vi "old_HWGlobalsToObject.vi"(7 "Select Layout":refnum<vi>, 8 "error in (no error)":errorcluster, 10 "Master AO Channel":T1, 11 "NI Card in":refnum<class "NI Card.lvclass">) -> (0 "error out":errorcluster, 3 "NI Card out":refnum<class "NI Card.lvclass">)   [LabVIEW 2013, in "NI Card.lvclass"]
uses:
  NI Card.lvclass
  NI Card.lvclass/NI Card.ctl
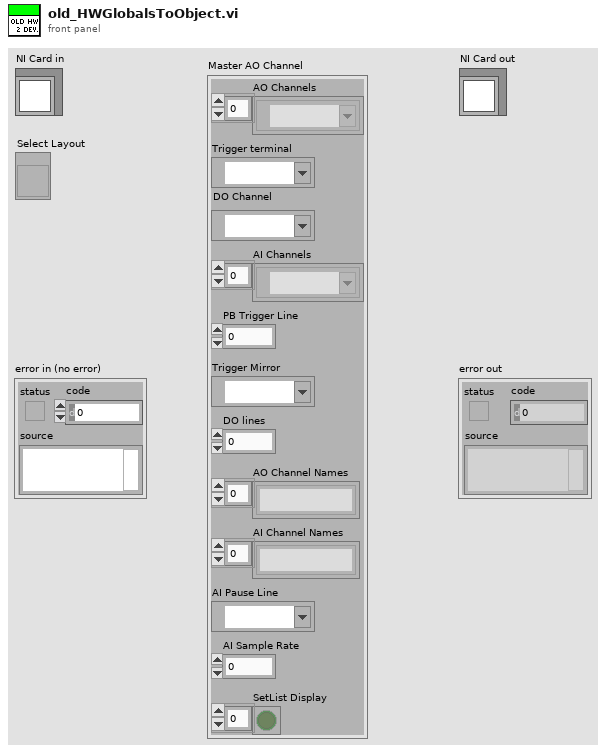
[diagram p1: front panel]
types:
  T1 = cluster{"AO Channels":refnum<k21>[], "Trigger terminal":tag, "DO Channel":refnum<k21>, "AI Channels":refnum<k21>[], "PB Trigger Line":u16, "Trigger Mirror":tag, "DO lines":i32, "AO Channel Names":string[], "AI Channel Names":string[], "AI Pause Line":tag, "AI Sample Rate":dbl, "SetList Display":bool[]}
  T2 = cluster{"DAQmx Global Channel":refnum<k21>, "String":string}
  T3 = cluster{"AI Pause Line":tag, "AI Sample Rate":dbl, "Trigger terminal":tag, "DO Channel":refnum<k21>, "Trigger Mirror":tag}
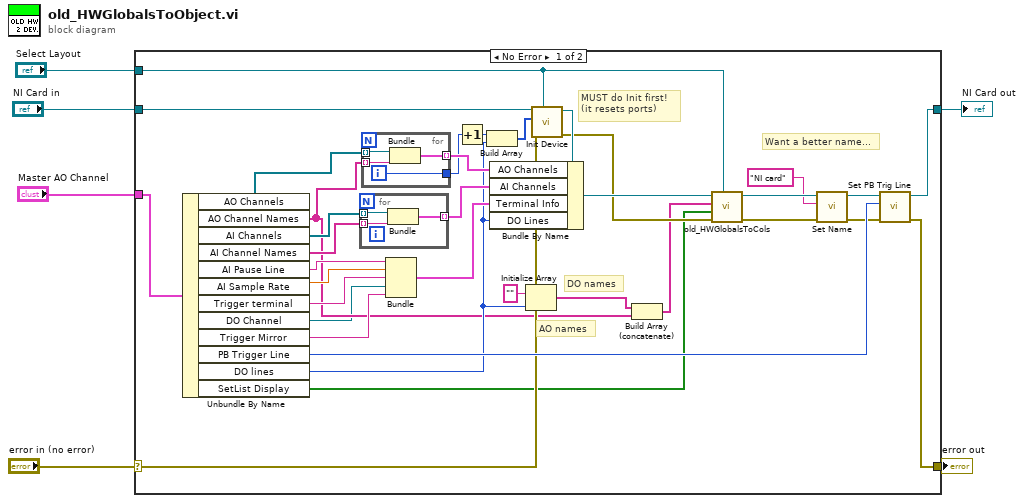
[diagram p0: block diagram]
diagram:
  n1 = case shown="No Error" "error in (no error)" {
    selector: "error in (no error)" -> [w27 w50]
    tunnel: [w31 w50] -> w5
    tunnel: [w30 w49] -> w4
    tunnel: "NI Card in" -> [w20 w49]
    tunnel: "Master AO Channel" -> [w41 _]
    tunnel: "Select Layout" -> [w17 _]
    frame No Error {
      # "Want a better name..."
      # "MUST do Init first! \n(it resets ports)"
      # "DO names"
      # "AO names"
      n2 = Unbundle By Name(w41) -> ("AO Channels"=w28:refnum<k21>[], "AO Channel Names"=w22:string[], "AI Channels"=w39:refnum<k21>[], "AI Channel Names"=w38:string[], "AI Pause Line"=w36:tag, "AI Sample Rate"=w35:dbl, "Trigger terminal"=w34:tag, "DO Channel"=w7:refnum<k21>, "Trigger Mirror"=w29:tag, "PB Trigger Line"=w32:u16, "DO lines"=w24:i32, "SetList Display"=w15:bool[])
      n3 = for {
        tunnel: w39 -> [w43] mode=indexing
        tunnel: w38 -> [w44] mode=indexing
        tunnel: [w42] -> w37 mode=indexing
        n4 = Bundle("DAQmx Global Channel"=w43, "String"=w44) -> (w42:T2)  [unwired: 1 in]
      }
      n5 = for {
        tunnel: w28 -> [w47] mode=indexing
        tunnel: w22 -> [w48] mode=indexing
        tunnel: [w46] -> w40 mode=indexing
        tunnel: [w45] -> w14
        i -> [w45]
        n6 = Bundle("DAQmx Global Channel"=w47, "String"=w48) -> (w46:T2)  [unwired: 1 in]
      }
      n7 = Bundle("AI Pause Line"=w36, "AI Sample Rate"=w35, "Trigger terminal"=w34, "DO Channel"=w7, "Trigger Mirror"=w29) -> (w33:T3)  [unwired: 1 in]
      n8 = Increment(x=w14) -> (x+1=w13:i32)
      n9 = Build Array(w13, w24) -> (w26:i32[])
      n10 = Initialize Array("", w24) -> (w23:string[])
      n11 = call-dynamic "Init Device.vi"("Layout Ref"=w17, "error in (no error)"=w27, "Chan# Array"=w26, "NI Card in"=w20) -> ("error out"=w18:errorcluster, "NI Card out"=w21:refnum<class "NI Card.lvclass">)  [unwired: 6 in]
      n12 = Bundle By Name(cluster=w21, "AO Channels"=w40, "AI Channels"=w37, "Terminal Info"=w33, "DO Lines"=w24) -> (w19:refnum<class "NI Card.lvclass">)
      n13 = Build Array (concatenate)(w23, w22) -> (w16:string[])
      n14 = call-dynamic "old_HWGlobalsToCols.vi"("Select Layout"=w17, "error in (no error)"=w18, "SetList Display"=w15, "Column Names"=w16, "Device in"=w19) -> ("error out"=w10:errorcluster, "Device out"=w12:refnum<class "NI Card.lvclass">)  [unwired: 5 in]
      n15 = call-dynamic "Set Name.vi"("error in (no error)"=w10, "Name"="NI card", "Device in"=w12) -> ("error out"=w9:errorcluster, "Device out"=w11:refnum<class "NI Card.lvclass">)  [unwired: 7 in]
      n16 = call-dynamic "Set PB Trig Line.vi"("error in (no error)"=w9, "PB Trigger Line"=w32, "Device in"=w11) -> ("error out"=w31:errorcluster, "Device out"=w30:refnum<class "NI Card.lvclass">)  [unwired: 7 in]
    }
    frame Error {
    }
  }
  "error out" <- w5
  "NI Card out" <- w4
